vi "Get Label Info Green.vi"() -> (5 "Label":string)   [LabVIEW 2013]
panel:
  in  "SCAN SERIAL NUMBER \nFROM LABEL":string
  in  "OK Button":bool
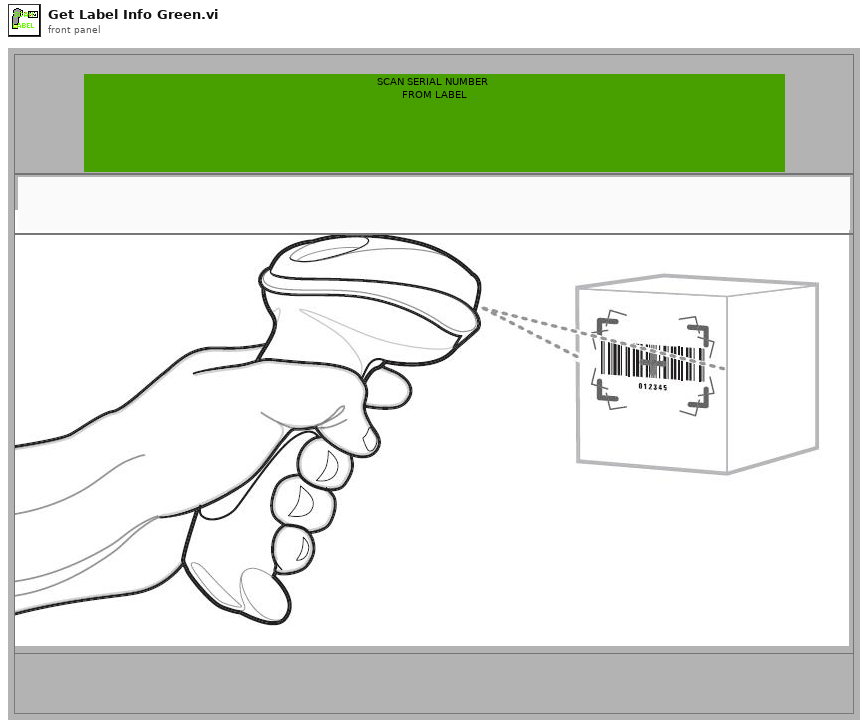
[diagram p1: front panel]
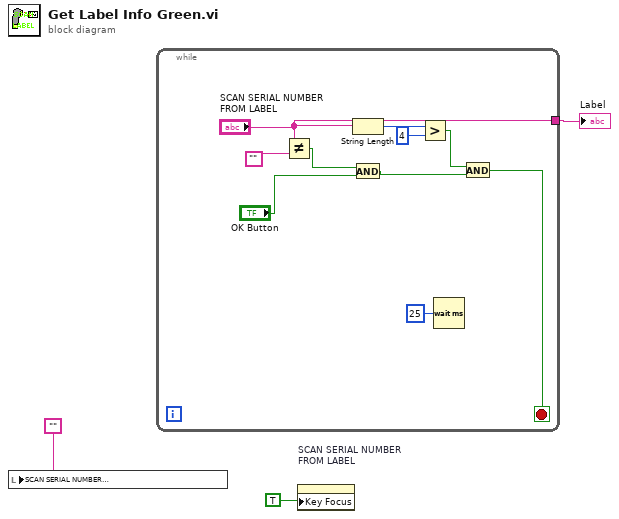
[diagram p0: block diagram]
diagram:
  n1 = local write "SCAN SERIAL NUMBER \nFROM LABEL"("") -> ()
  n2 = while {
    tunnel: ["SCAN SERIAL NUMBER \nFROM LABEL"] -> w1
    stop <- w6 stop-if-true
    n3 = Not Equal?(x="SCAN SERIAL NUMBER \nFROM LABEL", y="") -> (x != y?=w12:bool)
    n4 = String Length(string="SCAN SERIAL NUMBER \nFROM LABEL") -> (length=w10:i32)
    n5 = And(x=w12, y="OK Button") -> (x .and. y?=w7:bool)
    n6 = Greater?(x=w10, y=4) -> (0:w8:bool)
    n7 = Wait (ms)(milliseconds to wait=u32 25) -> ()  [unwired: 1 out]
    n8 = And(x=w8, y=w7) -> (x .and. y?=w6:bool)
  }
  "Label" <- w1
  n9 = property on="SCAN SERIAL NUMBER \nFROM LABEL" class="Str"("Key Focus"=TRUE) -> ()  [unwired: 2 in, 2 out]
